vi "prototype.vi"() -> ()   [LabVIEW 2015, in "lv-blog-interface-prototype.lvlib"]
uses:
  lv-blog-interface-prototype.lvlib
panel:
  in  "exit":bool
  in  "navigation":enum32{"tool", "build"}(radio) caption="Navigation"
  out "horizontal_progress_bar":dbl(slide) caption="Progress" scale=0.0..100.0
  out "tab_control":enum32{"Tool", "Build"}(tab)
  in  "select_project":bool
  in  "configure_tool":bool
  in  "dependencies":bool
  in  "open_dist_folder":bool
  in  "load_class":bool
  out "help_indicator":string="This space should be filled with something, possibly a general \"how to\" and some explanation in lieu of a help button? This may be an opportunity to add a logo if branding is desired"
  in  "configure_build":bool
  in  "build":bool
  in  "post":bool
  in  "start":bool
  in  "cancel":bool
  in  "targets_artifacts_tree":string[](tree)
  in  "status":string caption="Status"
  in  "git_commit_hash":string caption="Git Commit Hash"
  in  "version":string caption="Version"
  in  "project_file":string caption="Project"
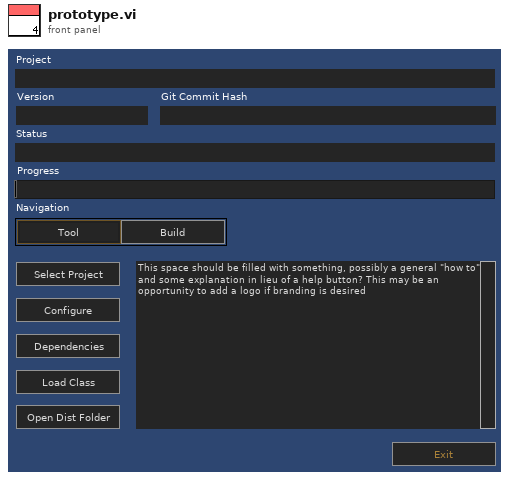
[diagram p1: front panel]
types:
  T1 = enum8{"Enabled", "Disabled", "Disabled and Grayed Out"}
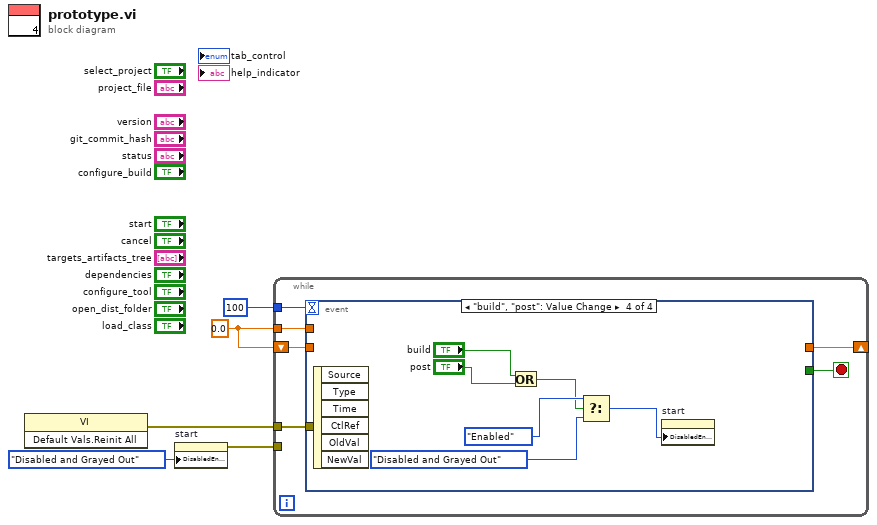
[diagram p0: block diagram]
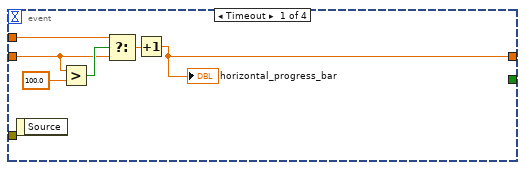
[diagram p2: hidden frame]
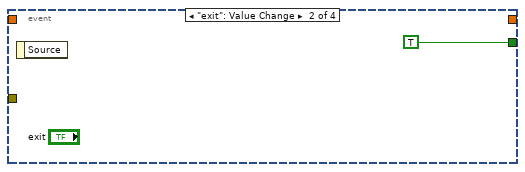
[diagram p3: hidden frame]
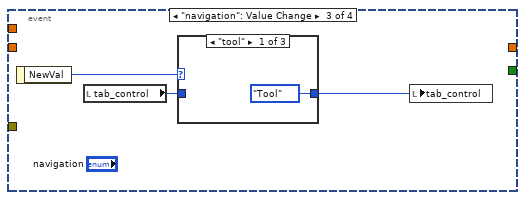
[diagram p4: hidden frame]
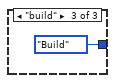
[diagram p6: hidden frame]
diagram:
  w4 = 0.0
  n1 = invoke class="VI" method="Default Vals.Reinit All"() -> (error out=w3:errorcluster)  [unwired: 3 in, 2 out]
  n2 = property on="start" class="Bool"("DisabledEnum"=T1."Disabled and Grayed Out" ("Disabled")) -> (error out=w1:errorcluster)  [unwired: 2 in, 1 out]
  n3 = while {
    tunnel: 100 -> [w10]
    shift-right: [w8] -> _
    shift-left: w4 -> [w9]
    tunnel: w4 -> [w7]
    tunnel: w3 -> [w6]
    tunnel: w1 -> [_]
    stop <- w11 stop-if-true
    n4 = event shown="[3] \"build\", \"post\": Value Change" {
      selector: _ -> [_ _ _ _]
      dyn-events: _ -> [_ _ _ _]
      timeout: w10 -> [_ _ _ _]
      tunnel: [_ TRUE _ _] -> w11
      tunnel: w9 -> [w14 _ _ _]
      tunnel: [w12 _ _ _] -> w8
      tunnel: w7 -> [w15 _ _ _]
      tunnel: w6 -> [_ _ _ _]
      event Timeout {
        n5 = event-data() -> ()  [unwired: 1 in, 1 out]
        n6 = Greater?(x=w14, y=100.0) -> (0:w16:bool)
        n7 = Select(t=w15, s=w16, f=w14) -> (s? t:f=w13:dbl)
        n8 = Increment(x=w13) -> (x+1=w12:dbl)
        "horizontal_progress_bar" <- w12
      }
      event "exit": Value Change {
        n9 = event-data() -> ()  [unwired: 1 in, 1 out]
      }
      event "navigation": Value Change {
        n10 = event-data() -> ("NewVal"=w21:enum32{"tool", "build"})  [unwired: 1 in]
        n11 = local read "tab_control"() -> (w20:enum32{"Tool", "Build"})
        n12 = case shown="\"tool\"" w21 {
          tunnel: w20 -> [_ w23 _]
          tunnel: [enum32{"Tool", "Build"}."Tool" ("tab_control") w23 enum32{"Tool", "Build"}."Build" ("tab_control")] -> w19
          frame "tool" {
          }
          frame Default {
          }
          frame "build" {
          }
        }
        n13 = local write "tab_control"(w19) -> ()
      }
      event "build", "post": Value Change {
        n14 = event-data() -> ()  [unwired: 1 in, 6 out]
        n15 = Or(x="build", y="post") -> (x .or. y?=w26:bool)
        n16 = Select(t=T1."Enabled" ("Disabled"), s=w26, f=T1."Disabled and Grayed Out" ("Disabled")) -> (s? t:f=w25:T1)
        n17 = property on="start" class="Bool"("DisabledEnum"=w25) -> ()  [unwired: 2 in, 2 out]
      }
    }
  }
